vi "PeripheralCoordinates.vi"(8 "Y End":sgl=10.0, 9 "Y Start":sgl, 10 "X End":sgl=10.0, 11 "X Start":sgl) -> (3 "Coordinate Array":sgl[][](array[numeric])=[[0.0, 0.0], [1.8, 0.0], [3.6, 0.0], [5.3999996, 0.0], [7.2, 0.0], [9.0, 0.0], [9.0, 2.0], [7.2, 2.0], [5.3999996, 2.0], [3.6, 2.0], [1.8, 2.0], [0.0, 2.0], [0.0, 4.0], [1.8, 4.0], [3.6, 4.0], [5.3999996, 4.0], [7.2, 4.0], [9.0, 4.0], [9.0, 6.0], [7.2, 6.0], [5.3999996, 6.0], [3.6, 6.0], [1.8, 6.0], [0.0, 6.0], [0.0, 8.0], [1.8, 8.0], [3.6, 8.0], [5.3999996, 8.0], [7.2, 8.0], [9.0, 8.0], [9.0, 10.0], [7.2, 10.0], [5.3999996, 10.0], [3.6, 10.0], [1.8, 10.0], [0.0, 10.0]])   [LabVIEW 2020]
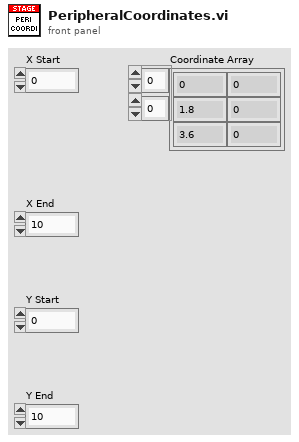
[diagram p1: front panel]
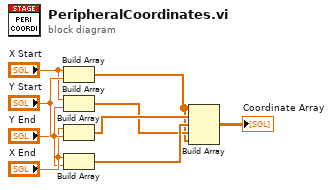
[diagram p0: block diagram]
diagram:
  n1 = Build Array("X Start", "Y Start") -> (w1:sgl[])
  n2 = Build Array("X Start", "Y End") -> (w2:sgl[])
  n3 = Build Array("X End", "Y Start") -> (w3:sgl[])
  n4 = Build Array("X End", "Y End") -> (w4:sgl[])
  n5 = Build Array(w1, w3, w4, w2, w1) -> (→"Coordinate Array":sgl[][])
